vi "Read_Write_ADAM_setup.vi"(3 "Mode":T1(ring)) -> ()   [LabVIEW 2015]
uses:
  ADAM Client/Sub VIs/ADAM Controls/Channel_State.ctl
  Anemometry/Anemometry Sub Vis/Globals/Constants_global.vi
  Anemometry/Anemometry Sub Vis/Globals/Gas_management_global.vi
  Exp conditions/EnFlo_Tun_Setup_global.vi
  ADAM_Global.vi
  Channel_Description_Global.vi
panel:
  out "Setup Filename":string
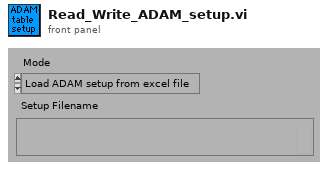
[diagram p1: front panel]
types:
  T1 = enum16{"Load ADAM setup from excel file", "Save ADAM setup to excel file"}
  T2 = typedef "Channel_State.ctl" = enum16{"On", "Off", "Always On", "Always Off"}
  T3 = typedef "Ch_description_ADAM.ctl" = cluster{"Ch Name":string, "Type":T4, "Function":T5, "Ch State":T2, "Calibration type":T6, "A":dbl, "B":dbl, "C":dbl, "D":dbl, "Comments":string, "Address":T7, "String":string, "Duty":u16}
  T4 = typedef "Module_type_ADAM.ctl" = string
  T5 = typedef "Function_ADAM.ctl" = enum16{"Analogue Input", "Digital Input", "Event counter", "Event rate", "Analogue Output", "Digital Output", "Relay Output"}
  T6 = typedef "Calib_type_ADAM.ctl" = enum16{"Raw", "Bx + A", "Cx^2 + Bx + A", "Dx^3 + Cx^2 + Bx + A", "In Band", "Hi-Tec Q", "Hi-Tec M_dot", "Text"}
  T7 = typedef "Address.ctl" = cluster{"Main":i32, "Ch.":i32, "Sub":i32, "Port Name":string}
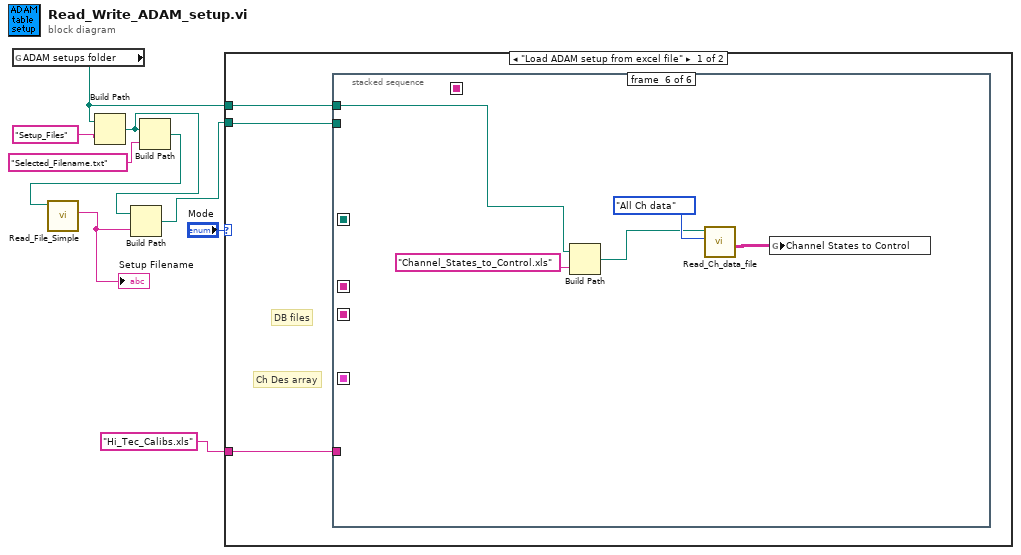
[diagram p0: block diagram]
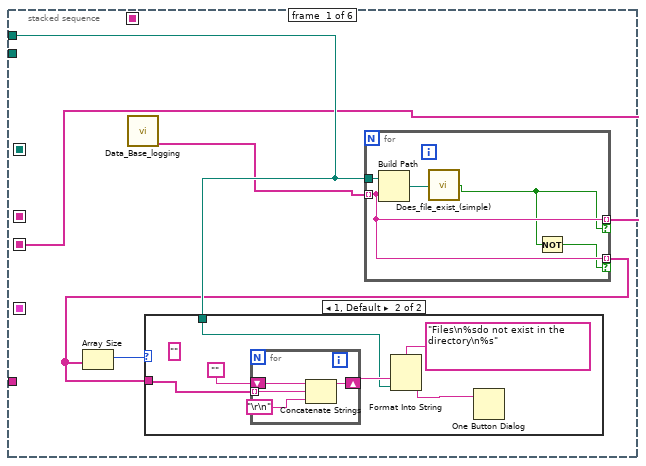
[diagram p2: hidden frame]
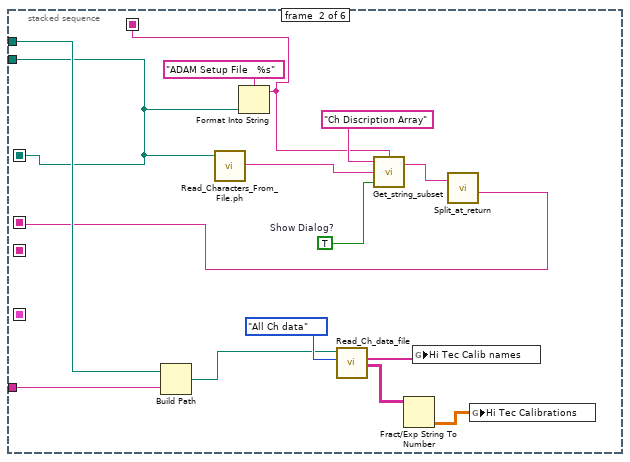
[diagram p4: hidden frame]
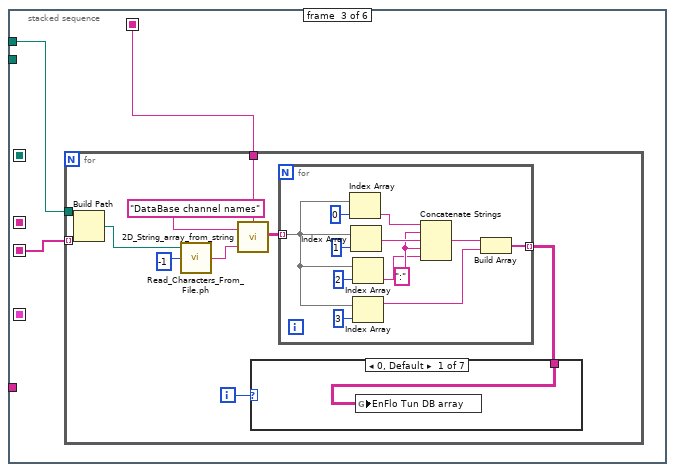
[diagram p5: hidden frame]
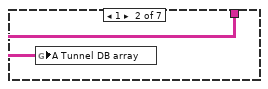
[diagram p6: hidden frame]
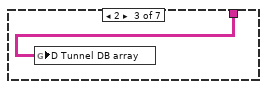
[diagram p7: hidden frame]
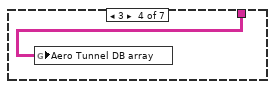
[diagram p8: hidden frame]
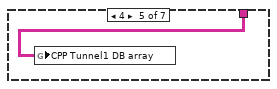
[diagram p9: hidden frame]
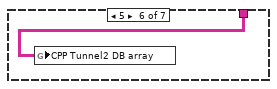
[diagram p10: hidden frame]
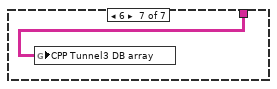
[diagram p11: hidden frame]
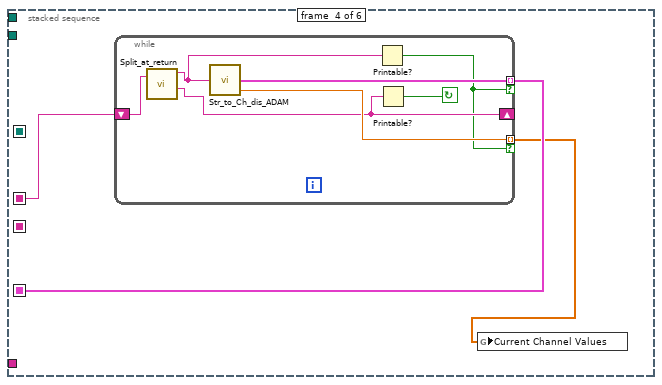
[diagram p12: hidden frame]
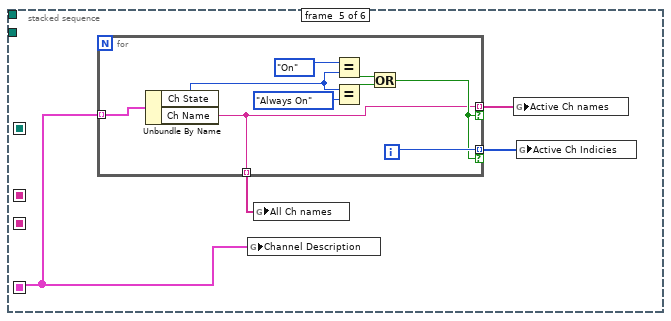
[diagram p13: hidden frame]
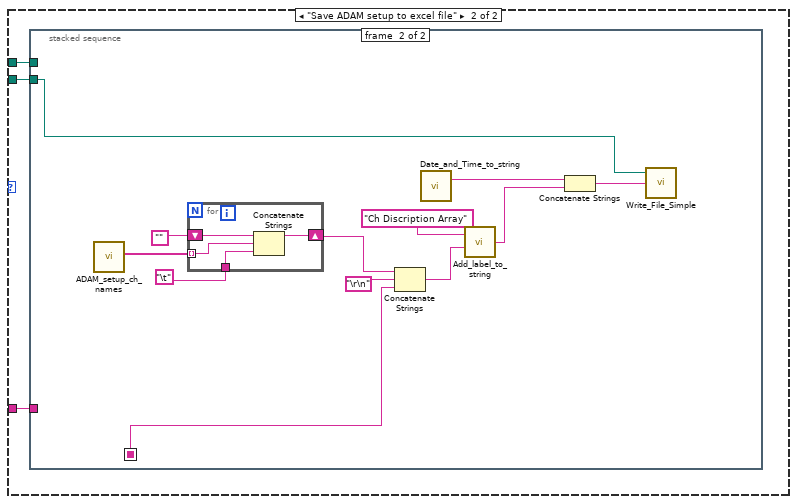
[diagram p14: hidden frame]
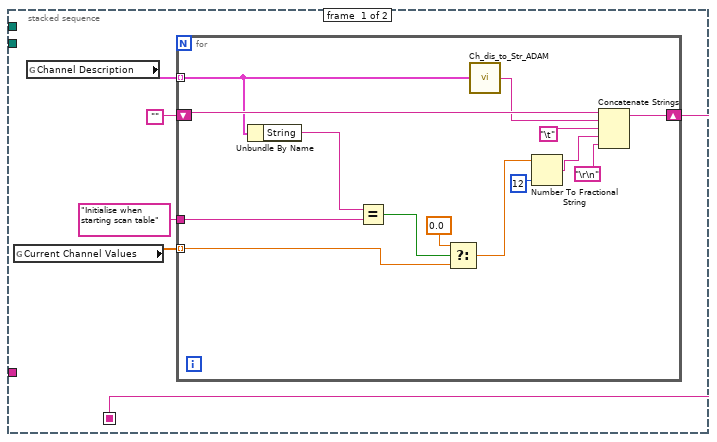
[diagram p15: hidden frame]
diagram:
  n1 = global read "Constants_global.vi" "ADAM setups folder"() -> (w8:path)
  n2 = Build Path(base path=w8, name or relative path="Setup_Files") -> (appended path=w4:path)
  n3 = Build Path(base path=w4, name or relative path="Selected_Filename.txt" ("Substring")) -> (appended path=w5:path)
  n4 = call "Read_File_Simple.vi"("Filename"=w5) -> ("string"=w3:string)  [unwired: 2 in, 7 out]
  "Setup Filename" <- w3
  n5 = Build Path(base path=w4, name or relative path=w3) -> (appended path=w2:path)
  n6 = case shown="\"Load ADAM setup from excel file\"" "Mode" {
    tunnel: w2 -> [w12 w110]
    tunnel: w8 -> [w11 w109]
    tunnel: "Hi_Tec_Calibs.xls" ("name or relative path") -> [w10 w108]
    frame "Load ADAM setup from excel file" {
      # "DB files"
      # "Ch Des array"
      n7 = stacked-sequence {
        seq-local: [_ w36 _ _ _ _] -> [_ _ _ w82 _ _]
        seq-local: [_ _ _ w81 _ _] -> [_ _ _ _ w93 _]
        seq-local: [_ w34 _ _ _ _] -> [_ _ _ _ _ _]
        seq-local: [w14 _ _ _ _ _] -> [_ _ w49 _ _ _]
        seq-local: [_ w33 _ _ _ _] -> [_ _ w48 _ _ _]
        tunnel: w12 -> [_ w34 _ _ _ _]
        tunnel: w11 -> [w16 w41 w50 _ _ w104]
        tunnel: w10 -> [_ w38 _ _ _ _]
        frame #0 {
          n8 = call "Data_Base_logging.vi"() -> ("DB Setup files"=w15:string[])  [unwired: 4 out]
          n9 = for {
            tunnel: w15 -> [w30] mode=indexing
            tunnel: w16 -> [w32]
            tunnel: [w30] -> w14 mode=indexing if=w29
            tunnel: [w30] -> w13 mode=indexing if=w28
            n10 = Build Path(base path=w32, name or relative path=w30) -> (appended path=w31:path)
            n11 = call "Does_file_exist_(simple).vi"("Pathname"=w31) -> ("exists?"=w29:bool)
            n12 = Not(x=w29) -> (.not. x?=w28:bool)
          }
          n13 = Array Size(array=w13) -> (size(s)=w17:i32)
          n14 = case shown="1, Default" w17 {
            tunnel: w16 -> [_ w20]
            tunnel: w13 -> [_ w22]
            frame 0 {
            }
            frame 1, Default {
              (unwired) ""
              n15 = for {
                shift-right: [w24] -> w21
                shift-left: "" -> [w27]
                tunnel: w22 -> [w25] mode=indexing
                n16 = Concatenate Strings(w27, w25, "\r\n") -> (w24:string)
              }
              n17 = Format Into String(format string="Files\n%sdo not exist in the directory\n%s" ("Format String"), w21, w20) -> (resulting string=w18:string)  [unwired: 2 in, 1 out]
              n18 = One Button Dialog(message=w18) -> ()  [unwired: 2 out]
            }
          }
        }
        frame #1 {
          w42 = TRUE  # Show Dialog?
          n19 = Build Path(base path=w41, name or relative path=w38) -> (appended path=w40:path)
          n20 = call "Read_Characters_From_File.ph.vi"("file path (dialog if empty)"=w34) -> ("character string"=w39:string)  [unwired: 1 in, 7 out]
          n21 = Format Into String(format string="ADAM Setup File   %s", w34) -> (resulting string=w33:string)  [unwired: 2 in, 1 out]
          n22 = call "Read_Ch_data_file.vi"("Output"=enum16{"All Ch data", "The last few rows"}."All Ch data", "Filename"=w40) -> ("Channel Values"=w44:string[][], "Merged Channels"=w45:string[])  [unwired: 3 in, 3 out]
          n23 = call "Get_string_subset.vi"("String Name"=w33, "Show Dialog?"=w42, "String to split"=w39, "File Label"="Ch Discription Array") -> ("Output string"=w37:string)  [unwired: 1 out]
          n24 = Fract/Exp String To Number(string=w44) -> (number=w43:dbl[][])  [unwired: 4 out]
          n25 = global write "Gas_management_global.vi" "Hi Tec Calib names"(w45) -> ()
          n26 = call "Split_at_return.vi"("String"=w37) -> ("after substring"=w36:string)  [unwired: 1 in, 3 out]
          n27 = global write "Gas_management_global.vi" "Hi Tec Calibrations"(w43) -> ()
        }
        frame #2 {
          n28 = for {
            tunnel: w50 -> [w54]
            tunnel: w49 -> [w53] mode=indexing
            tunnel: w48 -> [w51]
            i -> [w56]
            n29 = Build Path(base path=w54, name or relative path=w53) -> (appended path=w52:path)
            n30 = call "Read_Characters_From_File.ph.vi"("file path (dialog if empty)"=w52, "number of characters (all:-1)"=-1) -> ("character string"=w57:string)  [unwired: 7 out]
            n31 = call "2D_String_array_from_string.vi"("String Name"=w51, "Input string"=w57, "Array title"="DataBase channel names") -> ("2D data array"=w58:string[][])
            n32 = for {
              tunnel: w58 -> [w71] mode=indexing
              tunnel: [w69] -> w55 mode=indexing
              w74 = ":"
              n33 = Index Array(array=w71, index=0) -> (element=w76:string)
              n34 = Index Array(array=w71, index=1) -> (element=w75:string)
              n35 = Index Array(array=w71, index=2) -> (element=w73:string)
              n36 = Index Array(array=w71, index=3) -> (element=w70:string)
              n37 = Concatenate Strings(w76, w74, w75, w74, w73) -> (w68:string)
              n38 = Build Array(w68, w70) -> (w69:string[])
            }
            n39 = case shown="0, Default" w56 {
              tunnel: w55 -> [w61 w62 w63 w64 w65 w66 w67]
              frame 0, Default {
                n40 = global write "EnFlo_Tun_Setup_global.vi" "EnFlo Tun DB array"(w61) -> ()
              }
              frame 1 {
                n41 = global write "EnFlo_Tun_Setup_global.vi" "A Tunnel DB array"(w62) -> ()
              }
              frame 2 {
                n42 = global write "EnFlo_Tun_Setup_global.vi" "D Tunnel DB array"(w63) -> ()
              }
              frame 3 {
                n43 = global write "EnFlo_Tun_Setup_global.vi" "Aero Tunnel DB array"(w64) -> ()
              }
              frame 4 {
                n44 = global write "EnFlo_Tun_Setup_global.vi" "CPP Tunnel1 DB array"(w65) -> ()
              }
              frame 5 {
                n45 = global write "EnFlo_Tun_Setup_global.vi" "CPP Tunnel2 DB array"(w66) -> ()
              }
              frame 6 {
                n46 = global write "EnFlo_Tun_Setup_global.vi" "CPP Tunnel3 DB array"(w67) -> ()
              }
            }
          }
        }
        frame #3 {
          n47 = while {
            tunnel: [w88] -> w80 mode=indexing if=w83
            tunnel: [w89] -> w81 mode=indexing if=w83
            shift-left: w82 -> [w86]
            shift-right: [w87] -> _
            stop <- w84 continue-if-true
            n48 = call "Split_at_return.vi"("String"=w86) -> ("before substring"=w85:string, "after substring"=w87:string)  [unwired: 1 in, 2 out]
            n49 = call "Str_to_Ch_dis_ADAM.vi"("String Row"=w85) -> ("Value"=w88:dbl, "Ch Description"=w89:T3)  [unwired: 1 in, 2 out]
            n50 = Printable?(1:w85) -> (0:w83:bool)
            n51 = Printable?(1:w87) -> (0:w84:bool)
          }
          n52 = global write "ADAM_Global.vi" "Current Channel Values"(w80) -> ()
        }
        frame #4 {
          n53 = for {
            tunnel: w93 -> [w97] mode=indexing
            tunnel: [w94] -> w92 mode=indexing if=w95
            tunnel: [w96] -> w91 mode=indexing if=w95
            tunnel: [w94] -> w90 mode=indexing
            i -> [w96]
            n54 = Unbundle By Name(w97) -> ("Ch State"=w98:T2, "Ch Name"=w94:string)
            n55 = Equal?(x=Channel_State."On" ("Channel State"), y=w98) -> (x = y?=w100:bool)
            n56 = Equal?(x=w98, y=Channel_State."Always On" ("Channel State")) -> (x = y?=w99:bool)
            n57 = Or(x=w100, y=w99) -> (x .or. y?=w95:bool)
          }
          n58 = global write "Channel_Description_Global.vi" "Channel Description"(w93) -> ()
          n59 = global write "ADAM_Global.vi" "All Ch names"(w90) -> ()
          n60 = global write "ADAM_Global.vi" "Active Ch names"(w92) -> ()
          n61 = global write "ADAM_Global.vi" "Active Ch Indicies"(w91) -> ()
        }
        frame #5 {
          n62 = Build Path(base path=w104, name or relative path="Channel_States_to_Control.xls") -> (appended path=w106:path)
          n63 = call "Read_Ch_data_file.vi"("Output"=enum16{"All Ch data", "The last few rows"}."All Ch data", "Filename"=w106) -> ("Channel Values"=w103:string[][])  [unwired: 3 in, 4 out]
          n64 = global write "ADAM_Global.vi" "Channel States to Control"(w103) -> ()
        }
      }
    }
    frame "Save ADAM setup to excel file" {
      n65 = stacked-sequence {
        seq-local: [w114 _] -> [_ w134]
        tunnel: w110 -> [_ w131]
        tunnel: w109 -> [_ _]
        tunnel: w108 -> [_ _]
        frame #0 {
          n66 = global read "ADAM_Global.vi" "Current Channel Values"() -> (w113:dbl[])
          n67 = global read "Channel_Description_Global.vi" "Channel Description"() -> (w111:T3[])
          n68 = for {
            shift-right: [w116] -> w114
            shift-left: "" -> [w129]
            tunnel: w111 -> [w128] mode=indexing
            tunnel: w113 -> [w127] mode=indexing
            tunnel: "Initialise when starting scan table" ("y") -> [w126]
            n69 = Unbundle By Name(w128) -> ("String"=w119:string)
            n70 = Equal?(x=w119, y=w126) -> (x = y?=w118:bool)
            n71 = Select(t=0.0, s=w118, f=w127) -> (s? t:f=w120:dbl)
            n72 = call "Ch_dis_to_Str_ADAM.vi"("Ch Description"=w128) -> ("String Row"=w125:string)  [unwired: 4 out]
            n73 = Number To Fractional String(number=w120, precision (6)=i16 12) -> (F-format string=w121:string)  [unwired: 2 out]
            n74 = Concatenate Strings(w129, w125, "\t", w121, "\r\n") -> (w116:string)
          }
        }
        frame #1 {
          n75 = call "ADAM_setup_ch_names.vi"() -> ("Ch Names"=w133:string[])  [unwired: 1 out]
          n76 = for {
            shift-right: [w142] -> w132
            shift-left: "" -> [w145]
            tunnel: "\t" -> [w143]
            tunnel: w133 -> [w144] mode=indexing
            n77 = Concatenate Strings(w145, w144, w143) -> (w142:string)
          }
          n78 = Concatenate Strings(w132, "\r\n", w134) -> (w140:string)
          n79 = call "Date_and_Time_to_string.vi"() -> ("Date and time (spreadsheet)"=w139:string)
          n80 = call "Add_label_to_string.vi"("String to write"=w140, "File Label"="Ch Discription Array") -> ("Output string"=w138:string)
          n81 = Concatenate Strings(w139, w138) -> (w130:string)
          n82 = call "Write_File_Simple.vi"("character string"=w130, "file path"=w131) -> ()  [unwired: 1 in, 2 out]
        }
      }
    }
  }
